vi "template.vi"(11 "Statechart State":T1) -> (3 "Stop?":bool)   [LabVIEW 2010]
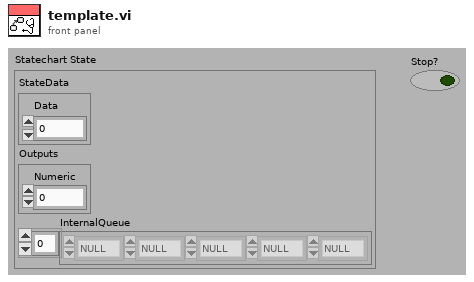
[diagram p1: front panel]
types:
  T1 = cluster{"StateData":cluster{"Data":i8}, "Outputs":cluster{"Numeric":i8}, "InternalQueue":enum16{"NULL"}[]}
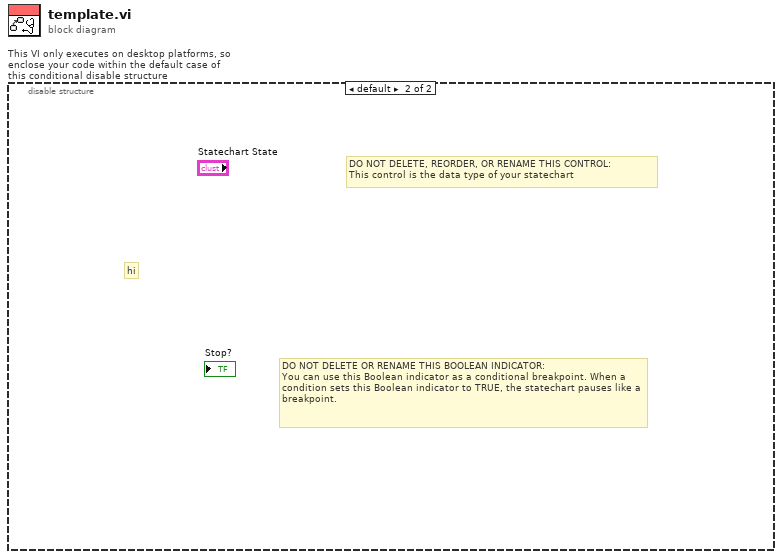
[diagram p0: block diagram]
diagram:
  n1 = disable-structure "This VI only executes on desktop platforms, so enclose your code within the default case of this conditional disable structure" shown="default" {
    frame condition #0 {
    }
    frame condition #1 (active) {
      # "hi"
      # "DO NOT DELETE OR RENAME THIS BOOLEAN INDICATOR: \nYou can use this Boolean indicator as a conditional breakpoint. When a condition sets this Boolean indicator to TRUE, the statechart pauses like a breakpoint."
      # "DO NOT DELETE, REORDER, OR RENAME THIS CONTROL: \nThis control is the data type of your statechart"
    }
  }
